vi "Impedance tube v0.8.vi"() -> ()   [LabVIEW 2021]
uses:
  <vilib>/express/express analysis/Spectral/Block/exnSpectralBlock spectral measurements RMS poly.vi
  <vilib>/express/express analysis/Spectral/Block/exnSpectralBlock spectral measurements RMS DDT.vi
  <vilib>/express/express arith-compare/Formula/XNode/ExpressFormulaBlockNode.xnode
  <vilib>/express/express analysis/Spectral/XNode/ExpressSpectralMeasurementsBlockNode.xnode
  <vilib>/Analysis/NI_AALPro.lvlib
panel:
  out "Probe":dbl[](graph)
  out "Rr":dbl[](graph)
  out "Absorption coeff":dbl[](graph)
  in  "number of samples":i32=2048
  out "MIC 2":dynamicdata(graph)
  out "MIC 2":dbl
  out "FFT1":dynamicdata(graph)
  out "MIC 1":dynamicdata(graph)
  out "MIC 1":dbl
  in  "stop (F)":bool
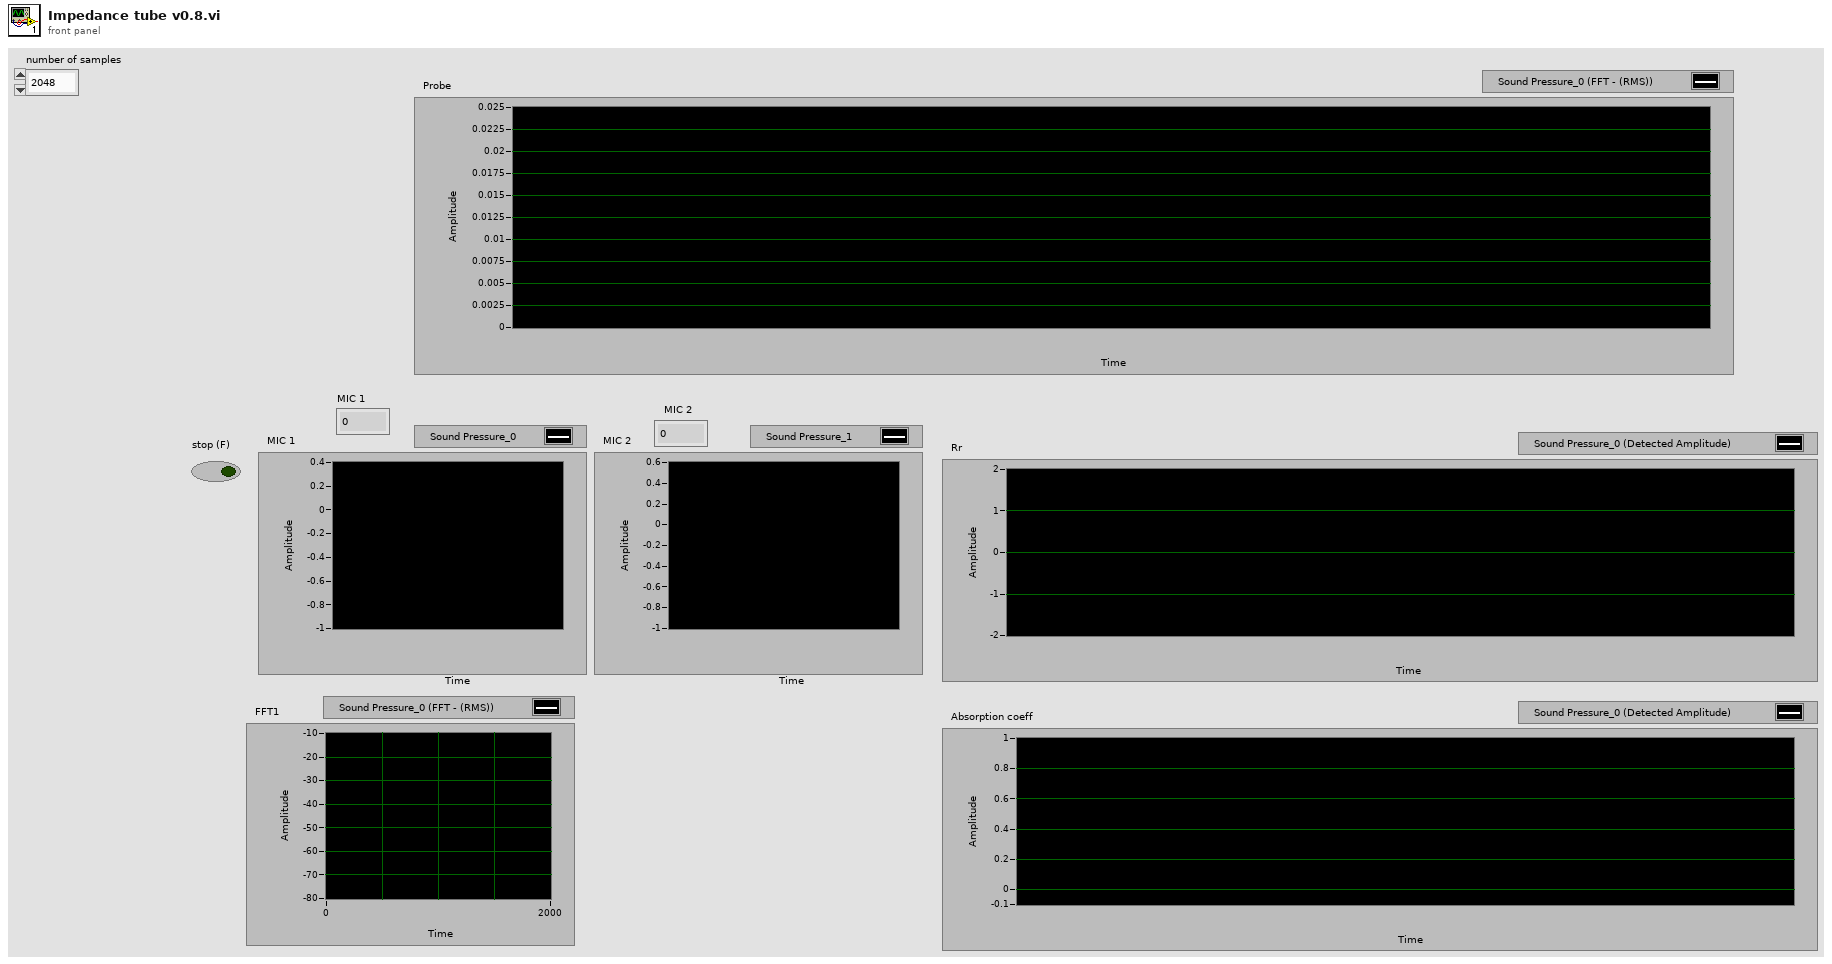
[diagram p1: front panel]
types:
  T1 = cluster{"averaging mode":u16, "weighting mode":u16, "number of averages":u32}
  T2 = cluster{"dB On (F)":bool, "unwrap phase (F)":bool, "convert to degree (F)":bool}
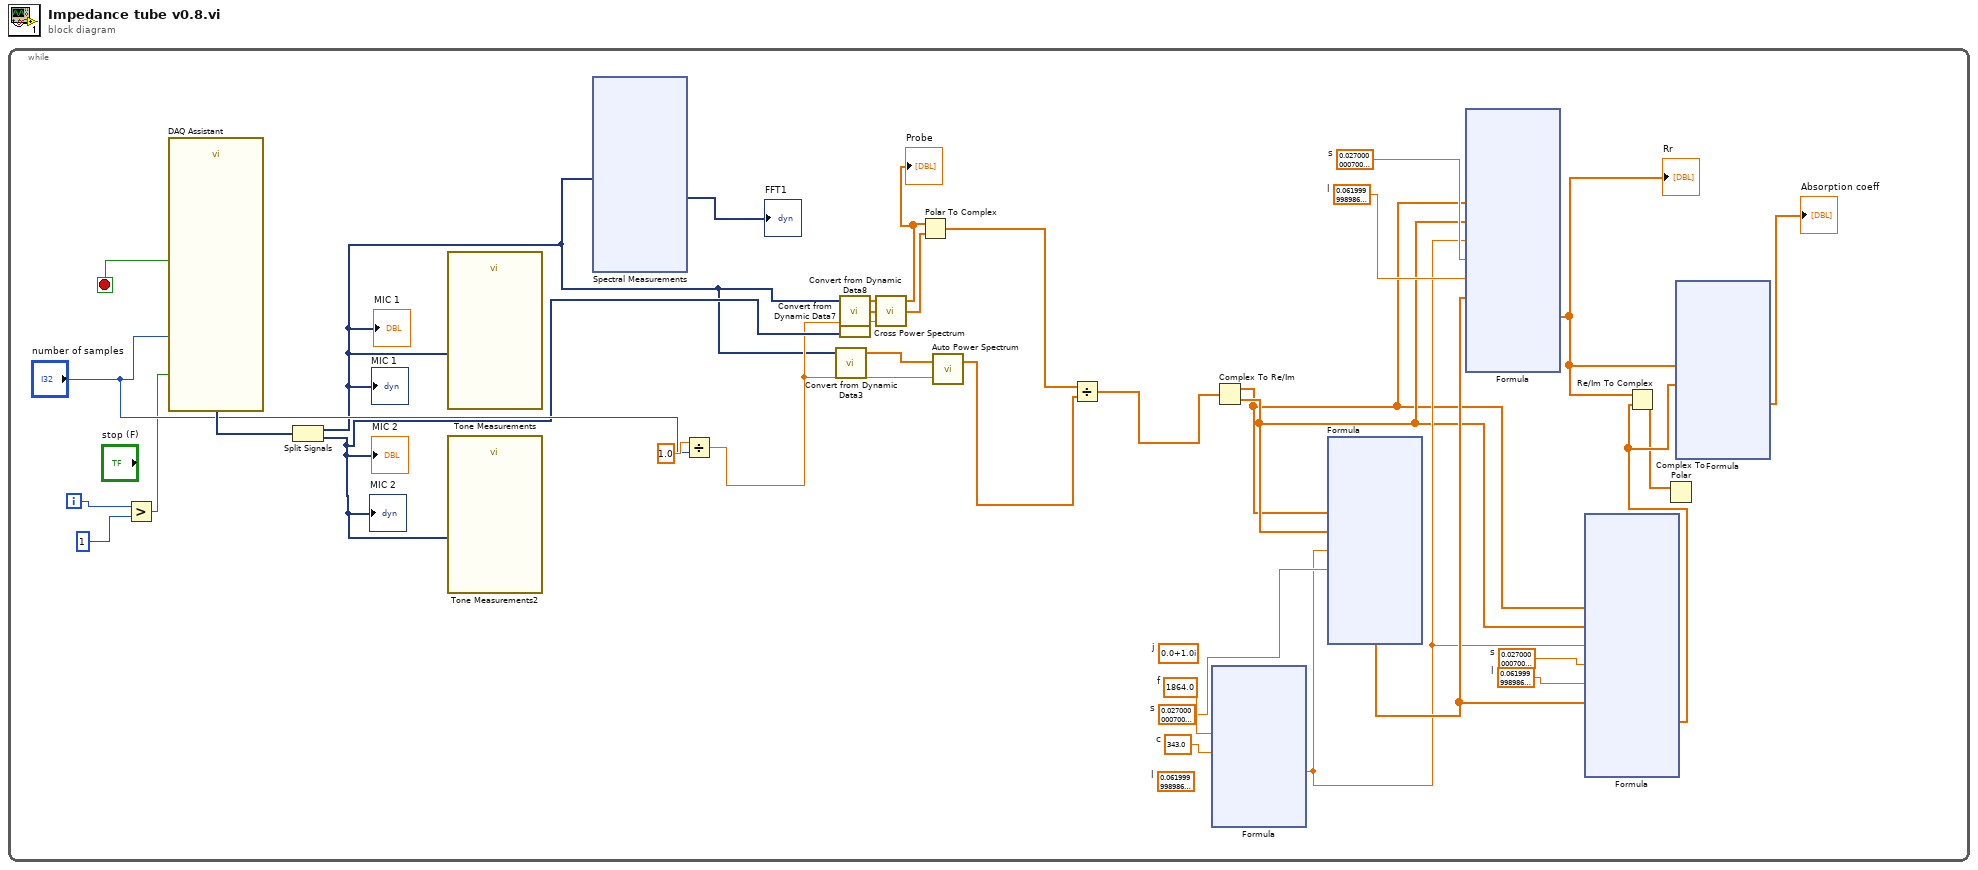
[diagram p0: block diagram]
diagram:
  n1 = while {
    i -> [w21]
    stop <- w34 stop-if-true
    w26 = sgl 0.062  # l
    w27 = sgl 0.027  # s
    w28 = sgl 0.062  # l
    w29 = sgl 0.027  # s
    (unwired) sgl 0.062  # l
    w32 = sgl 1864.0  # f
    w30 = sgl 0.027  # s
    w31 = sgl 343.0  # c
    (unwired) csg 0.0+1.0i  # j
    n2 = Greater?(x=w21, y=1) -> (0:w13:bool)
    n3 = call "DAQ Assistant"("number of samples"="number of samples", "stop (F)"=w13) -> ("data"=w33:dynamicdata, "stopped"=w34:bool)  [unwired: 14 in, 2 out]
    n4 = Split Signals(w33) -> (w5:dynamicdata, w10:dynamicdata)  [unwired: 2 in]
    "MIC 1" <- w5
    "MIC 1" <- w5
    "MIC 2" <- w10
    "MIC 2" <- w10
    n5 = call "Tone Measurements"("Signals"=w5) -> ()  [unwired: 8 in, 3 out]
    n6 = call "Tone Measurements2"("Signals"=w10) -> ()  [unwired: 8 in, 3 out]
    n7 = xnode "Spectral Measurements"("Signals"=w5) -> ("FFT - (RMS)"=→"FFT1":dynamicdata)  [unwired: 1 in, 2 out]
    n8 = Divide(x=1.0, y="number of samples") -> (x/y=w7:dbl)
    n9 = call "Convert from Dynamic Data3"("Dynamic Data Type"=w5) -> ("Array"=w4:dbl[])  [unwired: 3 in]
    n10 = call "Convert from Dynamic Data7"("Dynamic Data Type"=w5) -> ("Array"=w11:dbl[])  [unwired: 3 in]
    n11 = call "Convert from Dynamic Data8"("Dynamic Data Type"=w10) -> ("Array"=w9:dbl[])  [unwired: 3 in]
    n12 = call <vilib>:"Cross Power Spectrum.vi"("dt"=w7, "Signal Y (V)"=w9, "Signal X (V)"=w11) -> ("Cross Power XY Spectrum Phase (radians)"=w8:dbl[], "Cross Power XY Spectrum Mag (V^2rms)"=w6:dbl[])  [unwired: 1 out]
    "Probe" <- w6
    n13 = Polar To Complex(1:w8, 2:w6) -> (0:w3:cdb[])
    n14 = call <vilib>:"Auto Power Spectrum.vi"("dt"=w7, "Signal (V)"=w4) -> ("Power Spectrum (V^2 rms)"=w2:dbl[])  [unwired: 1 out]
    n15 = Divide(x=w3, y=w2) -> (x/y=w1:cdb[])
    n16 = xnode "Formula"("f"=w32, "c"=w31) -> ("Result"=w24:sgl)  [unwired: 1 in, 1 out]
    n17 = Complex To Re/Im(x + iy=w1) -> (x=w18:dbl[], y=w23:dbl[])
    n18 = xnode "Formula"("Hr"=w18, "Hi"=w23, "k"=w24, "s"=w30) -> ("Result"=w25:dbl[])  [unwired: 1 in, 1 out]
    n19 = xnode "Formula"("Hr"=w18, "Hi"=w23, "k"=w24, "s"=w29, "l"=w28, "D"=w25) -> ("Result"=w14:dbl[])  [unwired: 1 in, 1 out]
    "Rr" <- w14
    n20 = xnode "Formula"("Hr"=w18, "Hi"=w23, "k"=w24, "s"=w27, "l"=w26, "D"=w25) -> ("Result"=w22:dbl[])  [unwired: 1 in, 1 out]
    n21 = Re/Im To Complex(1:w22, 2:w14) -> (0:w19:cdb[])
    n22 = Complex To Polar(r * e^(i*theta)=w19) -> ()  [unwired: 2 out]
    n23 = xnode "Formula"("Rr"=w14, "Ri"=w22) -> ("Result"=→"Absorption coeff":dbl[])  [unwired: 1 in, 1 out]
  }
